vi "Red Stock.vi"   [LabVIEW 2019]
uses:
  Global Var.vi
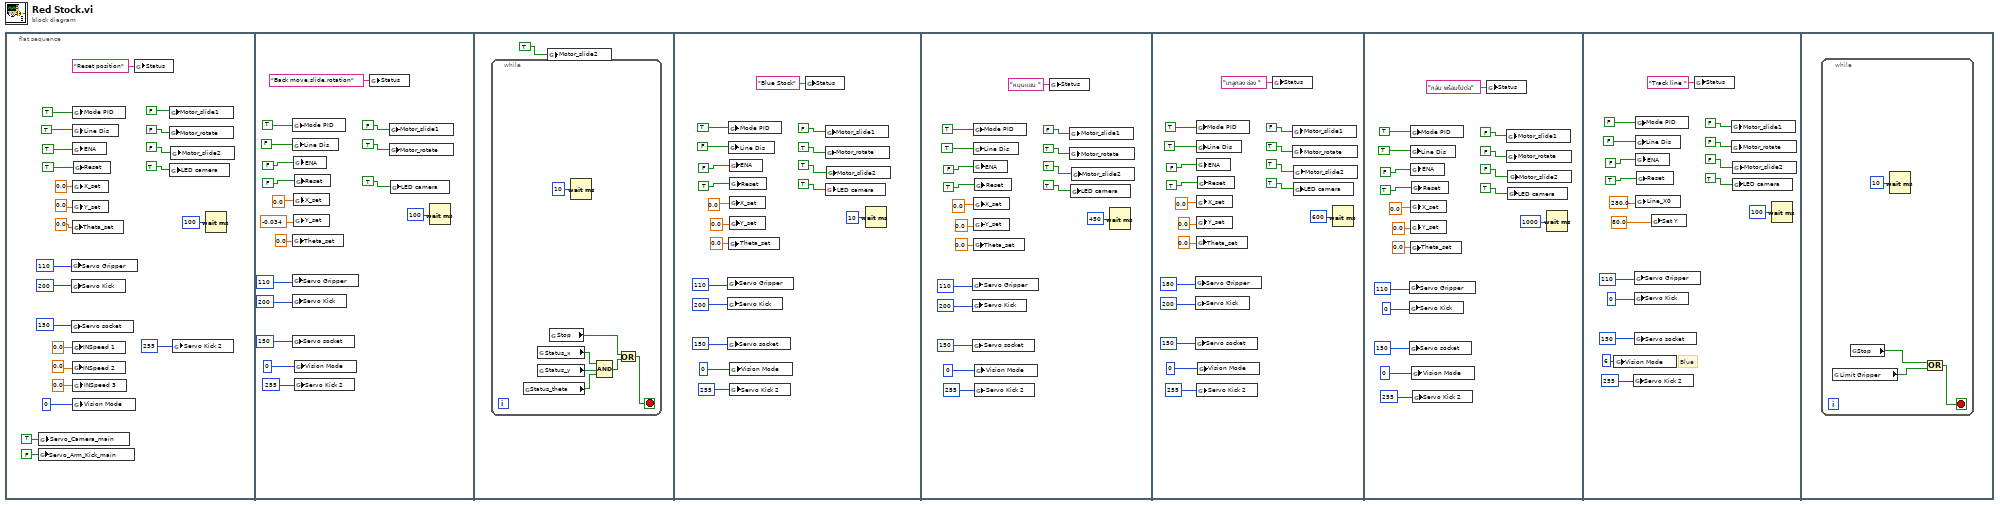
[diagram p0: block diagram]
diagram:
  n1 = flat-sequence {
    frame #0 {
      n2 = global write "Global Var.vi" "Servo_Arm_Kick_main"(FALSE ("Mode PID")) -> ()
      n3 = global write "Global Var.vi" "Servo_Camera_main"(TRUE ("Mode PID")) -> ()
      n4 = global write "Global Var.vi" "Servo Gripper"(u8 110 ("Servo Camera")) -> ()
      n5 = global write "Global Var.vi" "Servo Kick"(u8 200 ("Servo Camera")) -> ()
      n6 = global write "Global Var.vi" "Servo socket"(u8 150 ("Servo Camera")) -> ()
      n7 = global write "Global Var.vi" "Theta_set"(0.0 ("Theta_set")) -> ()
      n8 = global write "Global Var.vi" "INSpeed 1"(0.0 ("X_set")) -> ()
      n9 = global write "Global Var.vi" "INSpeed 2"(0.0 ("Y_set")) -> ()
      n10 = global write "Global Var.vi" "Mode PID"(TRUE ("Mode PID")) -> ()
      n11 = global write "Global Var.vi" "Line Dis"(TRUE ("Mode PID")) -> ()
      n12 = global write "Global Var.vi" "ENA"(TRUE ("ENA")) -> ()
      n13 = global write "Global Var.vi" "X_set"(0.0 ("X_set")) -> ()
      n14 = global write "Global Var.vi" "Y_set"(0.0 ("Y_set")) -> ()
      n15 = global write "Global Var.vi" "INSpeed 3"(0.0 ("Theta_set")) -> ()
      n16 = global write "Global Var.vi" "Vision Mode"(i16 0 ("Vision Mode")) -> ()
      n17 = global write "Global Var.vi" "Reset"(TRUE ("ENA")) -> ()
      n18 = global write "Global Var.vi" "Status"("Reset position" ("Status")) -> ()
      n19 = global write "Global Var.vi" "Motor_slide1"(FALSE ("Mode PID")) -> ()
      n20 = global write "Global Var.vi" "Motor_rotate"(FALSE ("ENA")) -> ()
      n21 = global write "Global Var.vi" "LED camera"(TRUE ("LED camera")) -> ()
      n22 = global write "Global Var.vi" "Motor_slide2"(FALSE ("ENA")) -> ()
      n23 = global write "Global Var.vi" "Servo Kick 2"(u8 255 ("Servo Camera")) -> ()
      n24 = Wait (ms)(milliseconds to wait=u32 100) -> ()  [unwired: 1 out]
    }
    frame #1 {
      n25 = global write "Global Var.vi" "Servo Gripper"(u8 110 ("Servo Camera")) -> ()
      n26 = global write "Global Var.vi" "Servo Kick"(u8 200 ("Servo Camera")) -> ()
      n27 = global write "Global Var.vi" "Servo socket"(u8 150 ("Servo Camera")) -> ()
      n28 = global write "Global Var.vi" "Mode PID"(TRUE ("Mode PID")) -> ()
      n29 = global write "Global Var.vi" "Line Dis"(FALSE ("Mode PID")) -> ()
      n30 = global write "Global Var.vi" "Theta_set"(0.0 ("Theta_set")) -> ()
      n31 = global write "Global Var.vi" "ENA"(FALSE ("ENA")) -> ()
      n32 = global write "Global Var.vi" "X_set"(0.0 ("X_set")) -> ()
      n33 = global write "Global Var.vi" "Y_set"(-0.034 ("Y_set")) -> ()
      n34 = global write "Global Var.vi" "Reset"(FALSE ("ENA")) -> ()
      n35 = global write "Global Var.vi" "Vision Mode"(i16 0 ("Vision Mode")) -> ()
      n36 = global write "Global Var.vi" "Servo Kick 2"(u8 255 ("Servo Camera")) -> ()
      n37 = global write "Global Var.vi" "Status"("Back move,slide,rotation" ("Status")) -> ()
      n38 = global write "Global Var.vi" "Motor_slide1"(FALSE ("Mode PID")) -> ()
      n39 = global write "Global Var.vi" "Motor_rotate"(TRUE ("ENA")) -> ()
      n40 = global write "Global Var.vi" "LED camera"(TRUE ("LED camera")) -> ()
      n41 = Wait (ms)(milliseconds to wait=u32 100) -> ()  [unwired: 1 out]
    }
    frame #2 {
      n42 = while {
        stop <- w44 stop-if-true
        n43 = global read "Global Var.vi" "Status_theta"() -> (w46:bool)
        n44 = global read "Global Var.vi" "Status_x"() -> (w47:bool)
        n45 = global read "Global Var.vi" "Status_y"() -> (w48:bool)
        n46 = global read "Global Var.vi" "Stop"() -> (w42:bool)
        n47 = Wait (ms)(milliseconds to wait=u32 10) -> ()  [unwired: 1 out]
        n48 = Compound Arithmetic op=AND(w47, w48, w46) -> (w43:bool)
        n49 = Or(x=w42, y=w43) -> (x .or. y?=w44:bool)
      }
      n50 = global write "Global Var.vi" "Motor_slide2"(TRUE ("ENA")) -> ()
    }
    frame #3 {
      n51 = global write "Global Var.vi" "Servo Gripper"(u8 110 ("Servo Camera")) -> ()
      n52 = global write "Global Var.vi" "Servo Kick"(u8 200 ("Servo Camera")) -> ()
      n53 = global write "Global Var.vi" "Servo socket"(u8 150 ("Servo Camera")) -> ()
      n54 = global write "Global Var.vi" "Mode PID"(TRUE ("Mode PID")) -> ()
      n55 = global write "Global Var.vi" "Line Dis"(FALSE ("Mode PID")) -> ()
      n56 = global write "Global Var.vi" "Theta_set"(0.0 ("Theta_set")) -> ()
      n57 = global write "Global Var.vi" "ENA"(FALSE ("ENA")) -> ()
      n58 = global write "Global Var.vi" "X_set"(0.0 ("X_set")) -> ()
      n59 = global write "Global Var.vi" "Y_set"(0.0 ("Y_set")) -> ()
      n60 = global write "Global Var.vi" "Reset"(TRUE ("ENA")) -> ()
      n61 = global write "Global Var.vi" "Vision Mode"(i16 0 ("Vision Mode")) -> ()
      n62 = global write "Global Var.vi" "Servo Kick 2"(u8 255 ("Servo Camera")) -> ()
      n63 = global write "Global Var.vi" "Status"("Blue Stock" ("Status")) -> ()
      n64 = global write "Global Var.vi" "Motor_slide1"(FALSE ("Mode PID")) -> ()
      n65 = global write "Global Var.vi" "Motor_rotate"(TRUE ("ENA")) -> ()
      n66 = global write "Global Var.vi" "LED camera"(TRUE ("LED camera")) -> ()
      n67 = global write "Global Var.vi" "Motor_slide2"(TRUE ("ENA")) -> ()
      n68 = Wait (ms)(milliseconds to wait=u32 10) -> ()  [unwired: 1 out]
    }
    frame #4 {
      n69 = global write "Global Var.vi" "Servo Gripper"(u8 110 ("Servo Camera")) -> ()
      n70 = global write "Global Var.vi" "Servo Kick"(u8 200 ("Servo Camera")) -> ()
      n71 = global write "Global Var.vi" "Servo socket"(u8 150 ("Servo Camera")) -> ()
      n72 = global write "Global Var.vi" "Mode PID"(TRUE ("Mode PID")) -> ()
      n73 = global write "Global Var.vi" "Line Dis"(TRUE ("Mode PID")) -> ()
      n74 = global write "Global Var.vi" "Theta_set"(0.0 ("Theta_set")) -> ()
      n75 = global write "Global Var.vi" "ENA"(FALSE ("ENA")) -> ()
      n76 = global write "Global Var.vi" "X_set"(0.0 ("X_set")) -> ()
      n77 = global write "Global Var.vi" "Y_set"(0.0 ("Y_set")) -> ()
      n78 = global write "Global Var.vi" "Reset"(TRUE ("ENA")) -> ()
      n79 = global write "Global Var.vi" "Vision Mode"(i16 0 ("Vision Mode")) -> ()
      n80 = global write "Global Var.vi" "Servo Kick 2"(u8 255 ("Servo Camera")) -> ()
      n81 = global write "Global Var.vi" "Status"("หมุนเเขน " ("Status")) -> ()
      n82 = global write "Global Var.vi" "Motor_slide1"(FALSE ("Mode PID")) -> ()
      n83 = global write "Global Var.vi" "Motor_rotate"(TRUE ("ENA")) -> ()
      n84 = global write "Global Var.vi" "LED camera"(TRUE ("LED camera")) -> ()
      n85 = global write "Global Var.vi" "Motor_slide2"(TRUE ("ENA")) -> ()
      n86 = Wait (ms)(milliseconds to wait=u32 450) -> ()  [unwired: 1 out]
    }
    frame #5 {
      n87 = global write "Global Var.vi" "Servo Gripper"(u8 180 ("Servo Camera")) -> ()
      n88 = global write "Global Var.vi" "Servo Kick"(u8 200 ("Servo Camera")) -> ()
      n89 = global write "Global Var.vi" "Servo socket"(u8 150 ("Servo Camera")) -> ()
      n90 = global write "Global Var.vi" "Mode PID"(TRUE ("Mode PID")) -> ()
      n91 = global write "Global Var.vi" "Line Dis"(TRUE ("Mode PID")) -> ()
      n92 = global write "Global Var.vi" "Theta_set"(0.0 ("Theta_set")) -> ()
      n93 = global write "Global Var.vi" "ENA"(FALSE ("ENA")) -> ()
      n94 = global write "Global Var.vi" "X_set"(0.0 ("X_set")) -> ()
      n95 = global write "Global Var.vi" "Y_set"(0.0 ("Y_set")) -> ()
      n96 = global write "Global Var.vi" "Servo Kick 2"(u8 255 ("Servo Camera")) -> ()
      n97 = global write "Global Var.vi" "Reset"(TRUE ("ENA")) -> ()
      n98 = global write "Global Var.vi" "Vision Mode"(i16 0 ("Vision Mode")) -> ()
      n99 = global write "Global Var.vi" "Status"("เทลูกลง ช่อง " ("Status")) -> ()
      n100 = global write "Global Var.vi" "Motor_slide1"(FALSE ("Mode PID")) -> ()
      n101 = global write "Global Var.vi" "Motor_rotate"(TRUE ("ENA")) -> ()
      n102 = global write "Global Var.vi" "LED camera"(TRUE ("LED camera")) -> ()
      n103 = global write "Global Var.vi" "Motor_slide2"(TRUE ("ENA")) -> ()
      n104 = Wait (ms)(milliseconds to wait=u32 600) -> ()  [unwired: 1 out]
    }
    frame #6 {
      n105 = global write "Global Var.vi" "Servo Gripper"(u8 110 ("Servo Camera")) -> ()
      n106 = global write "Global Var.vi" "Servo Kick"(u8 0 ("Servo Camera")) -> ()
      n107 = global write "Global Var.vi" "Servo socket"(u8 150 ("Servo Camera")) -> ()
      n108 = global write "Global Var.vi" "Mode PID"(TRUE ("Mode PID")) -> ()
      n109 = global write "Global Var.vi" "Line Dis"(TRUE ("Mode PID")) -> ()
      n110 = global write "Global Var.vi" "Theta_set"(0.0 ("Theta_set")) -> ()
      n111 = global write "Global Var.vi" "ENA"(FALSE ("ENA")) -> ()
      n112 = global write "Global Var.vi" "X_set"(0.0 ("X_set")) -> ()
      n113 = global write "Global Var.vi" "Y_set"(0.0 ("Y_set")) -> ()
      n114 = global write "Global Var.vi" "Reset"(TRUE ("ENA")) -> ()
      n115 = global write "Global Var.vi" "Vision Mode"(i16 0 ("Vision Mode")) -> ()
      n116 = global write "Global Var.vi" "Servo Kick 2"(u8 255 ("Servo Camera")) -> ()
      n117 = global write "Global Var.vi" "Status"("กลับ พร้อมไปต่อ" ("Status")) -> ()
      n118 = global write "Global Var.vi" "Motor_slide1"(FALSE ("Mode PID")) -> ()
      n119 = global write "Global Var.vi" "Motor_rotate"(FALSE ("ENA")) -> ()
      n120 = global write "Global Var.vi" "LED camera"(TRUE ("LED camera")) -> ()
      n121 = global write "Global Var.vi" "Motor_slide2"(FALSE ("ENA")) -> ()
      n122 = Wait (ms)(milliseconds to wait=u32 1000) -> ()  [unwired: 1 out]
    }
    frame #7 {
      # "Blue"
      n123 = global write "Global Var.vi" "Vision Mode"(i16 6 ("Vision Mode")) -> ()
      n124 = global write "Global Var.vi" "Servo Kick 2"(u8 255 ("Servo Camera")) -> ()
      n125 = global write "Global Var.vi" "Servo Gripper"(u8 110 ("Servo Camera")) -> ()
      n126 = global write "Global Var.vi" "Servo Kick"(u8 0 ("Servo Camera")) -> ()
      n127 = global write "Global Var.vi" "Servo socket"(u8 150 ("Servo Camera")) -> ()
      n128 = global write "Global Var.vi" "Mode PID"(FALSE ("Mode PID")) -> ()
      n129 = global write "Global Var.vi" "Line Dis"(FALSE ("Mode PID")) -> ()
      n130 = global write "Global Var.vi" "ENA"(FALSE ("ENA")) -> ()
      n131 = global write "Global Var.vi" "Line_X0"(280.0 ("Y_set")) -> ()
      n132 = global write "Global Var.vi" "Reset"(TRUE ("ENA")) -> ()
      n133 = global write "Global Var.vi" "Set Y"(80.0 ("Y_set")) -> ()
      n134 = global write "Global Var.vi" "Status"("Track line " ("Status")) -> ()
      n135 = global write "Global Var.vi" "Motor_slide1"(FALSE ("Mode PID")) -> ()
      n136 = global write "Global Var.vi" "Motor_rotate"(FALSE ("ENA")) -> ()
      n137 = global write "Global Var.vi" "LED camera"(TRUE ("LED camera")) -> ()
      n138 = global write "Global Var.vi" "Motor_slide2"(FALSE ("ENA")) -> ()
      n139 = Wait (ms)(milliseconds to wait=u32 100) -> ()  [unwired: 1 out]
    }
    frame #8 {
      n140 = while {
        stop <- w140 stop-if-true
        n141 = global read "Global Var.vi" "Limit Gripper"() -> (w138:bool)
        n142 = global read "Global Var.vi" "Stop"() -> (w139:bool)
        n143 = Wait (ms)(milliseconds to wait=u32 10) -> ()  [unwired: 1 out]
        n144 = Or(x=w139, y=w138) -> (x .or. y?=w140:bool)
      }
    }
  }
